vi "_io_parse_bin_data_header.vi"(5 "Timeout for chunked touts":i32=-1, 7 "Error when unrecognised header (T)":bool=TRUE, 8 "error in":errorcluster caption="error in (no error)", 9 "First read count (1)":i32=1, 11 "VISA resource name":refnum<visa-resource-name>) -> (0 "error out":errorcluster, 1 "Detected Data":T1, 2 "Size of the bin data":i64, 3 "VISA resource name out":refnum<visa-resource-name>, 4 "Unparsed read portion":string)   [LabVIEW 2020, in "Rohde&Schwarz RTx Oscilloscopes.lvlib" / "rsidr_core.lvlib"]
uses:
  rsidr_core.lvlib
  _type_Return_Data_Type.ctl
  type_Error_Codes.ctl
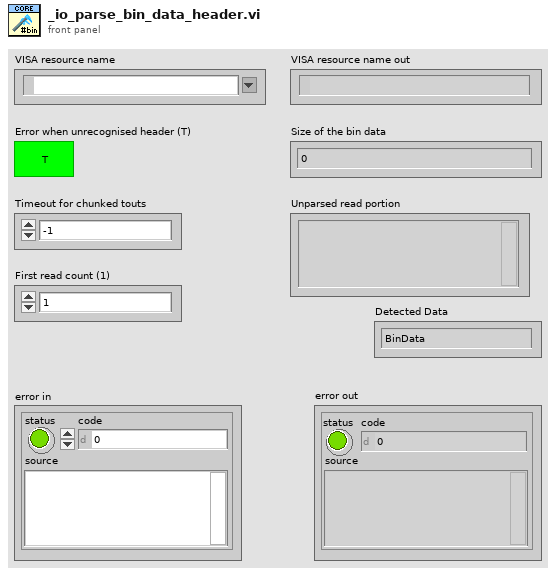
[diagram p1: front panel]
types:
  T1 = typedef "Rohde&Schwarz RTx Oscilloscopes.lvlib/rsidr_core.lvlib/_type_Return_Data_Type.ctl" = enum16{"BinData", "AsciiData", "EmptyAsciiData"}
  T2 = typedef "Rohde&Schwarz RTx Oscilloscopes.lvlib/rsidr_core.lvlib/type_Session_Data.ctl" = cluster{"IDN string":string, "Instrument FW":string, "Instr type":string, "Instr type for err. msg.":string, "Installed Options":string[], "Ignore Error Messages":string, "Logging params":variant, "OPC Timeout":i32, "VISA Timeout":i32, "STB Poll VISA Timeout":i32, "Additional Flags":i32, "Wait Before Read":i32, "Wait Before Write":i32, "Option String Flags":i32, "IO Segment Size":i64, "VISA Access Mode":T3, "Interface Type":T4, "OPC Wait Mode":T5, "Bin Float Number  Format":T6, "Bin Integer Number Format":T7, "Simulate":bool, "VXIcapable":bool, "Duplicate Session":bool, "Add LF to Write":bool, "Logging":bool, "Fast Sweep":bool, "Query Instrument Status":bool, "Check Range":bool, "Check Options":bool, "OPC-sync Attr Writes":bool, "OPC-sync Attr Queries":bool}
  T3 = typedef "Rohde&Schwarz RTx Oscilloscopes.lvlib/rsidr_core.lvlib/type_VisaAccessMode.ctl" = u16
  T4 = typedef "Rohde&Schwarz RTx Oscilloscopes.lvlib/rsidr_core.lvlib/type_InterfaceType.ctl" = enum16{"Unknown", "GPIB", "VXI", "GPIB_VXI", "ASRL", "PXI", "TCPIP", "USB", "SOCKET"}
  T5 = typedef "Rohde&Schwarz RTx Oscilloscopes.lvlib/rsidr_core.lvlib/type_OPC_Wait_Mode.ctl" = enum16{"STBpolling", "STBpollingSlow", "STBpollingSuperSlow", "ServiceRequest", "OPCquery"}
  T6 = typedef "Rohde&Schwarz RTx Oscilloscopes.lvlib/rsidr_core.lvlib/type_Binary_Float_Number_Format.ctl" = enum16{"Float_4_Bytes_Swapped", "Float_4_Bytes", "Double_8_Bytes_Swapped", "Double_8_Bytes"}
  T7 = typedef "Rohde&Schwarz RTx Oscilloscopes.lvlib/rsidr_core.lvlib/type_Binary_Integer_Number_Format.ctl" = enum16{"Int32_4_Bytes_Swapped", "Int32_4 Bytes", "Int16_2_Bytes_Swapped", "Int16_2_Bytes"}
  T8 = typedef "Rohde&Schwarz RTx Oscilloscopes.lvlib/rsidr_core.lvlib/type_Error_Codes.ctl" = enum16{"No_error", "VISA_err_ResourceNotFound", "VISA_err_Timeout", "VISA_warn_MoreDataAvailable", "RS_err_MissingCallback", "RS_err_InvalidAttribute", "RS_err_InvalidValue", "RS_err_UnknownResource", "RS_err_AlreadyInitialized", "RS_err_InstrumentStatus", "RS_err_BadRepCapName", "RS_err_TypesMismatch", "RS_err_ValueNotSupported", "RS_err_InvalidRngTable", "RS_err_IDqueryFail", "RS_err_UnexpResponse", "VISA_warn_ConfigNotLoaded", "RS_err_AttributeNotReadable", "RS_err_AttributeNotWritable", "RS_err_InstrumentType", "RS_err_InstrumentOption", "VISA_err_InvalidSize", "RS_err_ReliabilityIndicator", "VISA_warn_UnknownStatus", "VISA_warn_TermCharRead", "VISA_err_IO_error", "RS_err_FunctionNotSupported", "VISA_warn_QueueEmpty"}
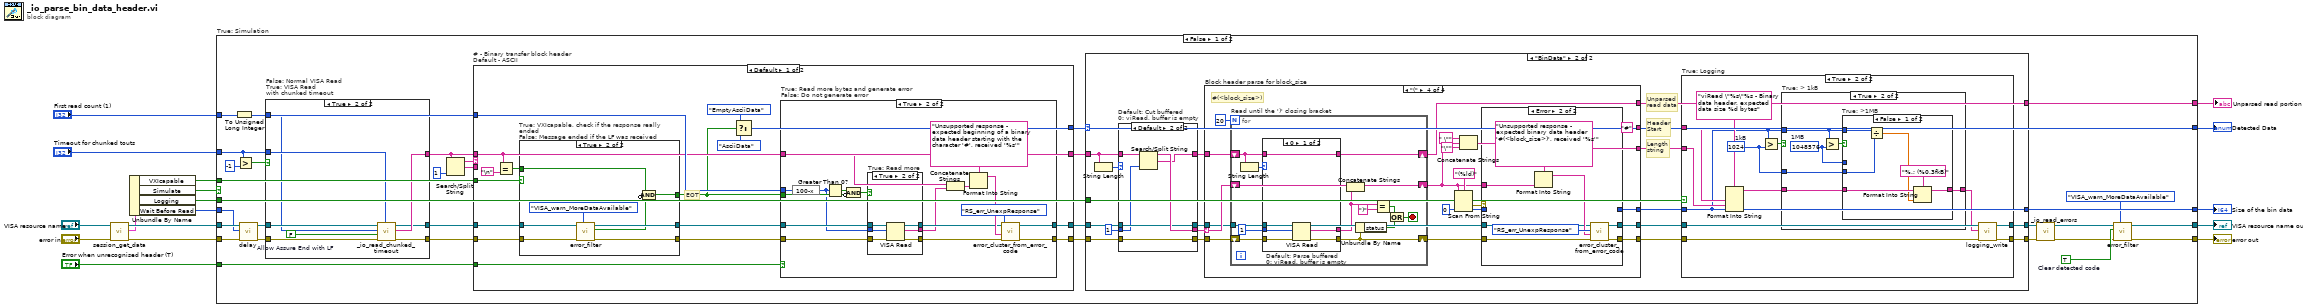
[diagram p0: block diagram]
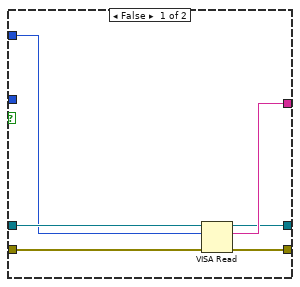
[diagram p2: hidden frame]
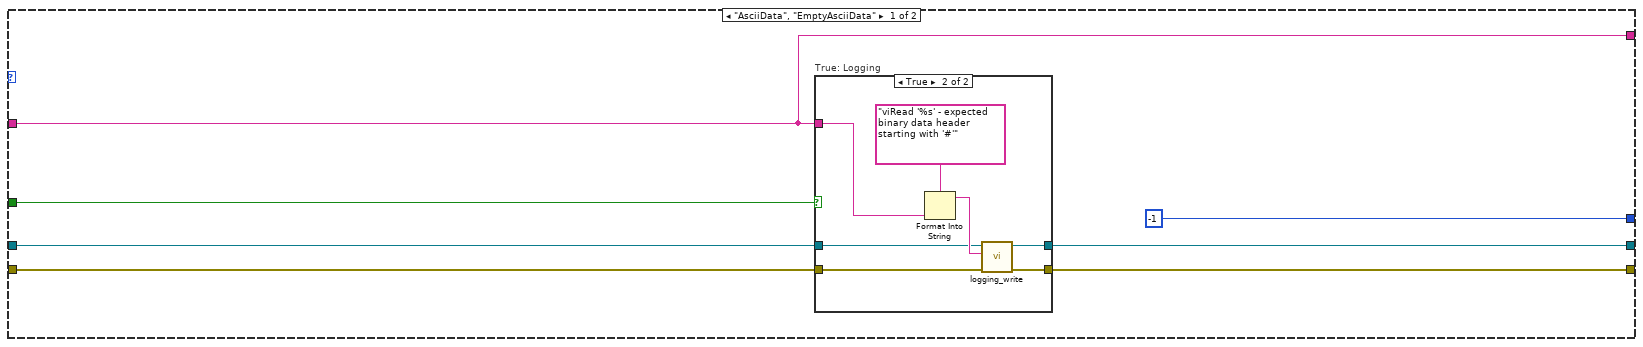
[diagram p3: hidden frame]
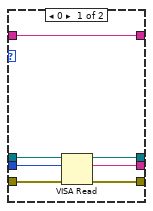
[diagram p5: hidden frame]
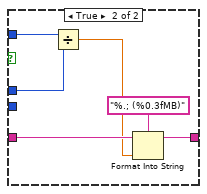
[diagram p8: hidden frame]
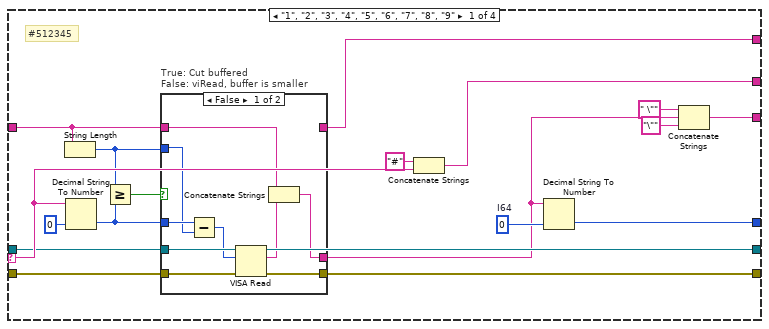
[diagram p9: hidden frame]
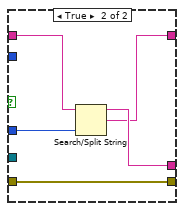
[diagram p10: hidden frame]
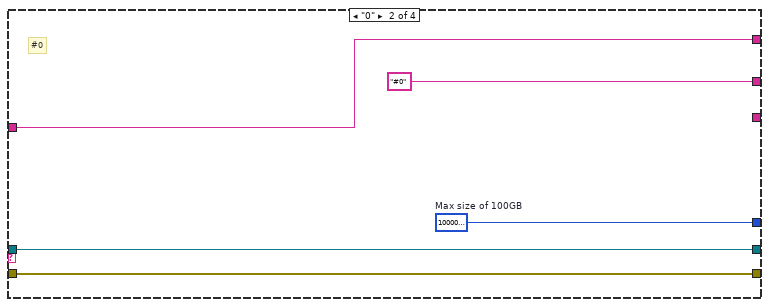
[diagram p11: hidden frame]
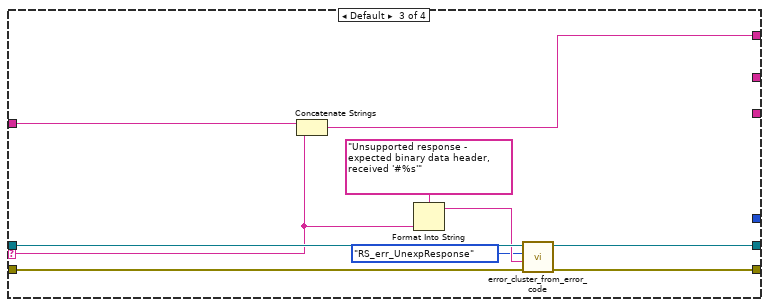
[diagram p12: hidden frame]
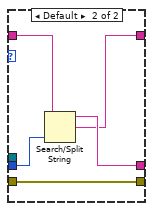
[diagram p13: hidden frame]
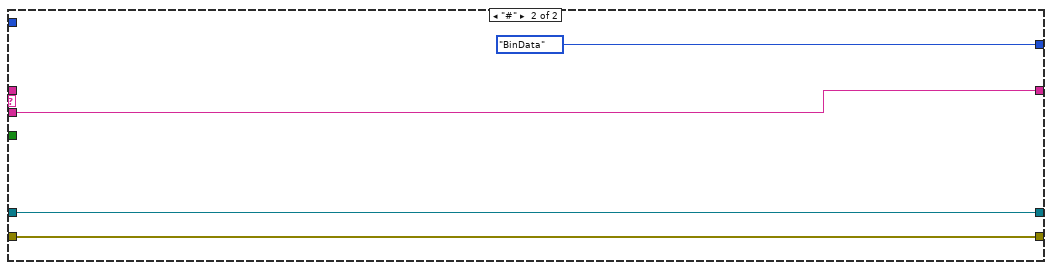
[diagram p18: hidden frame]
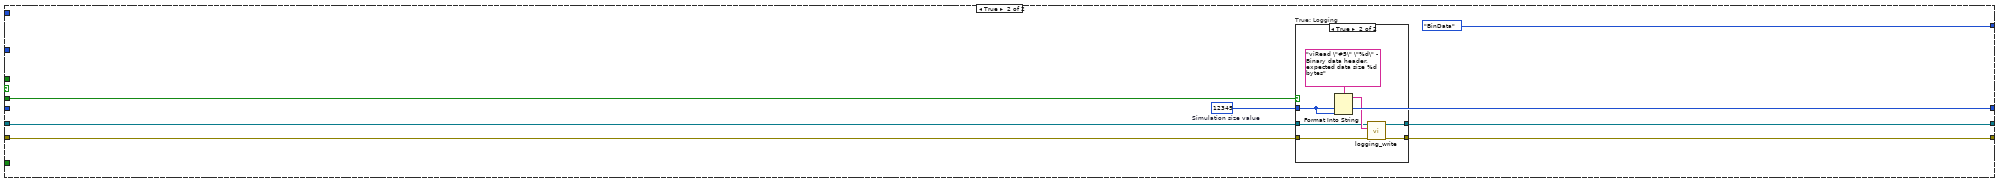
[diagram p19: hidden frame]
diagram:
  n1 = call "session_get_data.vi"("error in"="error in", "VISA resource name"="VISA resource name") -> ("error out"=w12:errorcluster, "Session User Data out"=w9:T2, "VISA resource name out"=w11:refnum<visa-resource-name>)  [unwired: 6 in, 1 out]
  n2 = Unbundle By Name(w9) -> ("VXIcapable"=w4:bool, "Simulate"=w10:bool, "Logging"=w8:bool, "Wait Before Read"=w5:i32)
  n3 = case "True: Simulation" shown="False" w10 {
    tunnel: [w47 w310] -> w17
    tunnel: w12 -> [w41 w309]
    tunnel: w11 -> [w40 w308]
    tunnel: [w32 w307] -> w16
    tunnel: [w31 w306] -> w15
    tunnel: w8 -> [w48 w305]
    tunnel: "Error when unrecognised header (T)" -> [w46 _]
    tunnel: [w20 _] -> w6
    tunnel: w5 -> [w37 _]
    tunnel: "Timeout for chunked touts" -> [w28 _]
    tunnel: w4 -> [w27 _]
    tunnel: "First read count (1)" -> [w22 _]
    tunnel: [w19 _type_Return_Data_Type."BinData" ("Detected Data")] -> w1
    frame False {
      w36 = TRUE  # Clear detected code
      n4 = To Unsigned Long Integer(number=w22) -> (unsigned 32bit integer=w18:u32)
      n5 = Greater?(x=w28, y=-1) -> (0:w29:bool)
      n6 = call "delay.vi"("error in"=w41, "Milliseconds to wait"=w37, "VISA resource name"=w40) -> ("error out"=w39:errorcluster, "VISA resource name out"=w38:refnum<visa-resource-name>)  [unwired: 7 in]
      n7 = case "False: Normal VISA Read\nTrue: VISA Read\nwith chunked timeout" shown="True" w29 {
        tunnel: [w56 w64] -> w50
        tunnel: [w55 w63] -> w23
        tunnel: [w54 w62] -> w45
        tunnel: w39 -> [w53 w61]
        tunnel: w38 -> [w52 w60]
        tunnel: w28 -> [_ w59]
        tunnel: w18 -> [w51 w58]
        frame False {
          n8 = VISA Read(VISA resource name=w52, byte count=w51, error in (no error)=w53) -> (VISA resource name out=w54:refnum<visa-resource-name>, read buffer=w55:string, error out=w56:errorcluster)  [unwired: 1 out]
        }
        frame True {
          w57 = FALSE  # Allow Assure End with LF
          n9 = call "_io_read_chunked_timeout.vi"("Timeout in"=w59, "error in"=w61, "Allow Assure End with LF"=w57, "Max bytes to read"=w58, "VISA resource name"=w60) -> ("error out"=w64:errorcluster, "Read buffer"=w63:string, "VISA resource name out"=w62:refnum<visa-resource-name>)  [unwired: 2 in, 2 out]
        }
      }
      n10 = Search/Split String(string=w23, offset (0)=1 ("length (rest)")) -> (substring before match=w25:string, match + rest of string=w24:string)  [unwired: 1 in, 1 out]
      n11 = case "# - Binary transfer block header\nDefault - ASCII" shown="Default" w25 {
        tunnel: w50 -> [w253 w303]
        tunnel: [w261 w303] -> w49
        tunnel: w46 -> [w259 _]
        tunnel: [w249 _type_Return_Data_Type."BinData" ("Detected Data")] -> w19
        tunnel: w45 -> [w252 w302]
        tunnel: [w260 w302] -> w44
        tunnel: w27 -> [w255 _]
        tunnel: w24 -> [_ w301]
        tunnel: w23 -> [w257 _]
        tunnel: w18 -> [w258 _]
        tunnel: [w257 w301] -> w21
        frame Default {
          # "EOT"
          n12 = Equal?(x=w257, y="\n") -> (x = y?=w254:bool)
          n13 = case "True: VXIcapable, check if the response really ended\nFalse: Message ended if the LF was received" shown="True" w255 {
            tunnel: w254 -> [w262 w267]
            tunnel: w253 -> [w264 w272]
            tunnel: w252 -> [w263 w271]
            tunnel: [w263 w270] -> w251
            tunnel: [w264 w269] -> w250
            tunnel: [w262 w265] -> w248
            frame False {
            }
            frame True {
              n14 = call "error_filter.vi"("Error Enum in"=type_Error_Codes."VISA_warn_MoreDataAvailable", "error in"=w272, "VISA resource name"=w271) -> ("error out"=w269:errorcluster, "Code Detected"=w266:bool, "VISA resource name out"=w270:refnum<visa-resource-name>)  [unwired: 6 in]
              n15 = Compound Arithmetic op=AND(w267, invert w266) -> (w265:bool)
            }
          }
          n16 = Select(t=_type_Return_Data_Type."EmptyAsciiData" ("Detected Data"), s=w248, f=_type_Return_Data_Type."AsciiData" ("Detected Data")) -> (s? t:f=w249:T1)
          n17 = case "True: Read more bytes and generate error\nFalse: Do not generate error" shown="True" w259 {
            tunnel: w250 -> [w274 w288]
            tunnel: [w274 w284] -> w261
            tunnel: w251 -> [w273 w287]
            tunnel: [w273 w283] -> w260
            tunnel: w257 -> [_ w280]
            tunnel: w258 -> [_ w276]
            tunnel: w248 -> [_ w279]
            frame False {
            }
            frame True {
              n18 = expression code="100-x"(w276) -> (w275:u32)
              n19 = Greater Than 0?(x=w275) -> (x > 0?=w277:bool)
              n20 = Compound Arithmetic op=AND(w277, invert w279) -> (w278:bool)
              n21 = case "True: Read more" shown="True" w278 {
                tunnel: w288 -> [w292 w299]
                tunnel: w287 -> [w293 w298]
                tunnel: [w292 w297] -> w286
                tunnel: [w293 w296] -> w285
                tunnel: [_ w295] -> w282
                tunnel: w275 -> [_ w294]
                frame False {
                }
                frame True {
                  n22 = VISA Read(VISA resource name=w298, byte count=w294, error in (no error)=w299) -> (VISA resource name out=w296:refnum<visa-resource-name>, read buffer=w295:string, error out=w297:errorcluster)  [unwired: 1 out]
                }
              }
              n23 = Concatenate Strings(w280, w282) -> (w281:string)
              n24 = Format Into String(format string="Unsupported response - expected beginning of a binary data header starting with the character '#', received '%s'" ("error message (\"\")"), w281) -> (resulting string=w289:string)  [unwired: 2 in, 1 out]
              n25 = call "error_cluster_from_error_code.vi"("error in"=w286, "Error Message (\"\")"=w289, "Error Enum in"=type_Error_Codes."RS_err_UnexpResponse", "VISA resource name"=w285) -> ("error out"=w284:errorcluster, "VISA resource name out"=w283:refnum<visa-resource-name>)  [unwired: 6 in]
            }
          }
        }
        frame "#" {
        }
      }
      n26 = case shown="\"BinData\"" w19 {
        tunnel: w49 -> [w70 w98]
        tunnel: w44 -> [w69 w94]
        tunnel: [w68 w93] -> w43
        tunnel: [w67 w92] -> w42
        tunnel: w48 -> [w66 w91]
        tunnel: w21 -> [w65 w82]
        tunnel: [i64 -1 ("default value 1") w88] -> w47
        tunnel: [w65 w81] -> w20
        frame "AsciiData", "EmptyAsciiData" {
          n27 = case "True: Logging" shown="True" w66 {
            tunnel: w70 -> [w72 w78]
            tunnel: w69 -> [w73 w77]
            tunnel: [w72 w76] -> w68
            tunnel: [w73 w75] -> w67
            tunnel: w65 -> [_ w74]
            frame False {
            }
            frame True {
              n28 = Format Into String(format string="viRead '%s' - expected binary data header starting with '#'" ("String to write"), w74) -> (resulting string=w79:string)  [unwired: 2 in, 1 out]
              n29 = call "logging_write.vi"("error in"=w78, "String to write"=w79, "VISA resource name"=w77) -> ("error out"=w76:errorcluster, "VISA resource name out"=w75:refnum<visa-resource-name>)  [unwired: 7 in]
            }
          }
        }
        frame "BinData" {
          # "Unparsed\nread data"
          # "Length\nstring"
          # "Header\nStart"
          n30 = String Length(string=w82) -> (length=w85:i32)
          n31 = case "Default: Cut buffered\n0: viRead, buffer is empty" shown="Default" w85 {
            tunnel: w98 -> [w105 w108]
            tunnel: [w104 w108] -> w97
            tunnel: [w103 w110] -> w96
            tunnel: [w102 w107] -> w95
            tunnel: w94 -> [w101 w107]
            tunnel: w82 -> [w99 w111]
            tunnel: [w99 w109] -> w84
            tunnel: u32 1 ("byte count (0)") -> [w100 w106]
            frame 0 {
              n32 = VISA Read(VISA resource name=w101, byte count=w100, error in (no error)=w105) -> (VISA resource name out=w102:refnum<visa-resource-name>, read buffer=w103:string, error out=w104:errorcluster)  [unwired: 1 out]
            }
            frame Default {
              n33 = Search/Split String(string=w111, offset (0)=w106) -> (substring before match=w110:string, match + rest of string=w109:string)  [unwired: 1 in, 1 out]
            }
          }
          n34 = case "Block header parse for block_size" shown="\"(\"" w96 {
            selector: w96 -> [w157 _ w181 w208]
            tunnel: w97 -> [w148 w180 w188 w209]
            tunnel: w95 -> [w149 w179 w187 w195]
            tunnel: [w161 w178 _ w200] -> w88
            tunnel: [w148 w180 w186 w202] -> w86
            tunnel: [w149 w179 w185 w194] -> w87
            tunnel: w84 -> [w153 w177 w189 w193]
            tunnel: [w158 "#0" _ "#"] -> w90
            tunnel: [w156 _ _ w197] -> w89
            tunnel: [w146 w177 w182 w192] -> w81
            frame "1", "2", "3", "4", "5", "6", "7", "8", "9" {
              w160 = i64 0  # I64
              # "#512345"
              n35 = String Length(string=w153) -> (length=w150:i32)
              n36 = Decimal String To Number(string=w157, default (0L)=0 ("default (0 I32)")) -> (number=w152:i32)  [unwired: 1 in, 1 out]
              n37 = Greater Or Equal?(x=w150, y=w152) -> (x >= y?=w151:bool)
              n38 = case "True: Cut buffered\nFalse: viRead, buffer is smaller" shown="False" w151 {
                tunnel: w148 -> [w170 w174]
                tunnel: [w169 w174] -> _
                tunnel: [w162 w175] -> w147
                tunnel: w149 -> [w168 _]
                tunnel: w152 -> [w167 w173]
                tunnel: w153 -> [w163 w172]
                tunnel: [_ w171] -> w146
                tunnel: w150 -> [w166 _]
                frame False {
                  n39 = Subtract(x=w167, y=w166) -> (x-y=w165:i32)
                  n40 = VISA Read(VISA resource name=w168, byte count=w165, error in (no error)=w170) -> (read buffer=w164:string, error out=w169:errorcluster)  [unwired: 2 out]
                  n41 = Concatenate Strings(w163, w164) -> (w162:string)
                }
                frame True {
                  n42 = Search/Split String(string=w172, offset (0)=w173) -> (substring before match=w175:string, match + rest of string=w171:string)  [unwired: 1 in, 1 out]
                }
              }
              n43 = Concatenate Strings("#" ("string"), w157) -> (w158:string)
              n44 = Decimal String To Number(string=w147, default (0L)=w160) -> (number=w161:i64)  [unwired: 1 in, 1 out]
              n45 = Concatenate Strings(" \"" ("string"), w147, "\"" ("string")) -> (w156:string)
            }
            frame "0" {
              w178 = i64 100000000000  # Max size of 100GB
              # "#0"
            }
            frame Default {
              n46 = Concatenate Strings(w189, w181) -> (w182:string)
              n47 = Format Into String(format string="Unsupported response - expected binary data header, received '#%s'" ("error message (\"\")"), w181) -> (resulting string=w184:string)  [unwired: 2 in, 1 out]
              n48 = call "error_cluster_from_error_code.vi"("error in"=w188, "Error Message (\"\")"=w184, "Error Enum in"=type_Error_Codes."RS_err_UnexpResponse", "VISA resource name"=w187) -> ("error out"=w186:errorcluster, "VISA resource name out"=w185:refnum<visa-resource-name>)  [unwired: 6 in]
            }
            frame "(" {
              # "#(<block_size>)"
              n49 = for "Read until the ')' closing bracket" {
                N: 20 -> [_]
                tunnel: w195 -> [w216]
                shift-right: [w222] -> w199
                shift-left: w208 -> [w223]
                shift-right: [w211] -> w204
                shift-left: w209 -> [w217]
                shift-right: [w212] -> w192
                shift-left: w193 -> [w213]
                stop <- w218 stop-if-true
                n50 = String Length(string=w213) -> (length=w214:i32)
                n51 = case "Default: Parse buffered\n0: viRead, buffer is empty" shown="0" w214 {
                  tunnel: w217 -> [w229 w233]
                  tunnel: [w228 w233] -> w211
                  tunnel: [w227 w234] -> w210
                  tunnel: w216 -> [w226 _]
                  tunnel: u32 1 ("byte count (0)") -> [w225 w232]
                  tunnel: w213 -> [w224 w231]
                  tunnel: [w224 w230] -> w212
                  frame 0 {
                    n52 = VISA Read(VISA resource name=w226, byte count=w225, error in (no error)=w229) -> (read buffer=w227:string, error out=w228:errorcluster)  [unwired: 2 out]
                  }
                  frame Default {
                    n53 = Search/Split String(string=w231, offset (0)=w232) -> (substring before match=w234:string, match + rest of string=w230:string)  [unwired: 1 in, 1 out]
                  }
                }
                n54 = Concatenate Strings(w223, w210) -> (w222:string)
                n55 = Unbundle By Name(w211) -> ("status"=w220:bool)
                n56 = Equal?(x=w210, y=")") -> (x = y?=w219:bool)
                n57 = Or(x=w219, y=w220) -> (x .or. y?=w218:bool)
              }
              n58 = Scan From String(format string="(%ld)", input string=w199, default 1=i64 0 ("default value 1")) -> (error out=w205:errorcluster, output 1=w201:i64)  [unwired: 2 in, 2 out]
              n59 = Concatenate Strings(" \"" ("string"), w199, "\"" ("string")) -> (w197:string)
              n60 = case shown="Error" w205 {
                tunnel: w204 -> [w236 w242]
                tunnel: w199 -> [_ w244]
                tunnel: [w236 w243] -> w202
                tunnel: w201 -> [w237 _]
                tunnel: [w237 _] -> w200
                tunnel: w195 -> [w235 w239]
                tunnel: [w235 w238] -> w194
                frame No Error {
                }
                frame Error {
                  n61 = Format Into String(format string="Unsupported response - expected binary data header  '#(<block_size>)', received '%s'" ("error message (\"\")"), w244) -> (resulting string=w240:string)  [unwired: 2 in, 1 out]
                  n62 = call "error_cluster_from_error_code.vi"("error in"=w242, "Error Message (\"\")"=w240, "Error Enum in"=type_Error_Codes."RS_err_UnexpResponse", "VISA resource name"=w239) -> ("error out"=w243:errorcluster, "VISA resource name out"=w238:refnum<visa-resource-name>)  [unwired: 6 in]
                }
              }
            }
          }
          n63 = case "True: Logging" shown="True" w91 {
            tunnel: w86 -> [w112 w125]
            tunnel: w87 -> [w113 w124]
            tunnel: [w112 w123] -> w93
            tunnel: [w113 w122] -> w92
            tunnel: w90 -> [_ w120]
            tunnel: w89 -> [_ w119]
            tunnel: w88 -> [_ w117]
            frame False {
            }
            frame True {
              w114 = i64 1024  # 1kB
              n64 = Format Into String(format string="viRead \"%s\"%s - Binary data header, expected data size %d bytes" ("String to write"), w120, w119, w117) -> (resulting string=w116:string)  [unwired: 2 in, 1 out]
              n65 = Greater?(x=w117, y=w114) -> (0:w118:bool)
              n66 = case "True: > 1kB" shown="True" w118 {
                tunnel: w117 -> [_ w131]
                tunnel: w116 -> [w126 w130]
                tunnel: [w126 w129] -> w115
                tunnel: w114 -> [_ w127]
                frame False {
                }
                frame True {
                  w128 = i64 1048576  # 1MB
                  n67 = Greater?(x=w131, y=w128) -> (0:w132:bool)
                  n68 = case "True: >1MB" shown="False" w132 {
                    tunnel: w131 -> [w135 w141]
                    tunnel: w130 -> [w137 w143]
                    tunnel: [w136 w142] -> w129
                    tunnel: w128 -> [_ w139]
                    tunnel: w127 -> [w133 _]
                    frame False {
                      n69 = Divide(x=w135, y=w133) -> (x/y=w134:dbl)
                      n70 = Format Into String(format string="%.; (%0.3fkB)", initial string=w137, w134) -> (resulting string=w136:string)  [unwired: 1 in, 1 out]
                    }
                    frame True {
                      n71 = Divide(x=w141, y=w139) -> (x/y=w140:dbl)
                      n72 = Format Into String(format string="%.; (%0.3fMB)", initial string=w143, w140) -> (resulting string=w142:string)  [unwired: 1 in, 1 out]
                    }
                  }
                }
              }
              n73 = call "logging_write.vi"("error in"=w125, "String to write"=w115, "VISA resource name"=w124) -> ("error out"=w123:errorcluster, "VISA resource name out"=w122:refnum<visa-resource-name>)  [unwired: 7 in]
            }
          }
        }
      }
      n74 = call "_io_read_errors.vi"("error in"=w43, "VISA resource name"=w42) -> ("error out"=w34:errorcluster, "VISA resource name out"=w33:refnum<visa-resource-name>)  [unwired: 8 in]
      n75 = call "error_filter.vi"("Error Enum in"=type_Error_Codes."VISA_warn_MoreDataAvailable", "error in"=w34, "Clear detected code (F)"=w36, "VISA resource name"=w33) -> ("error out"=w32:errorcluster, "VISA resource name out"=w31:refnum<visa-resource-name>)  [unwired: 5 in, 1 out]
    }
    frame True {
      w310 = i64 12345  # Simulation size value
      n76 = case "True: Logging" shown="True" w305 {
        tunnel: w309 -> [w311 w317]
        tunnel: w308 -> [w312 w316]
        tunnel: [w311 w315] -> w307
        tunnel: [w312 w314] -> w306
        tunnel: w310 -> [_ w313]
        frame False {
        }
        frame True {
          n77 = Format Into String(format string="viRead \"#5\" \"%d\" - Binary data header, expected data size %d bytes" ("String to write"), w313, w313) -> (resulting string=w318:string)  [unwired: 2 in, 1 out]
          n78 = call "logging_write.vi"("error in"=w317, "String to write"=w318, "VISA resource name"=w316) -> ("error out"=w315:errorcluster, "VISA resource name out"=w314:refnum<visa-resource-name>)  [unwired: 7 in]
        }
      }
    }
  }
  "error out" <- w16
  "VISA resource name out" <- w15
  "Size of the bin data" <- w17
  "Unparsed read portion" <- w6
  "Detected Data" <- w1
